vi "gfitsio-read-column-i32-scalar.vi"(7 "column":string, 8 "error in (no error)":errorcluster, 9 "row":i32, 11 "gfits refnum":T1) -> (0 "error out":errorcluster, 2 "data":i32, 3 "dup gfits refnum":T1)   [LabVIEW 2022 SP3, in "gfitsio.lvlib"]
doc: "Read elements from an ASCII or binary table column."
uses:
  gfitsio.lvlib
  gfitsio-refnum.ctl
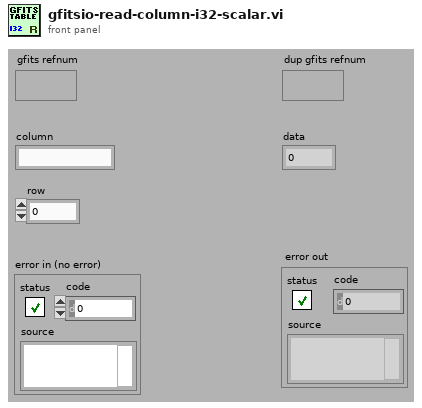
[diagram p1: front panel]
types:
  T1 = typedef "gfitsio.lvlib/gfitsio-refnum.ctl" = refnum<k1>
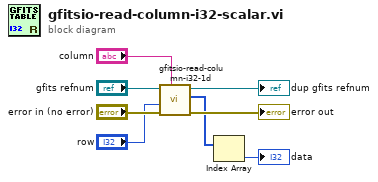
[diagram p0: block diagram]
diagram:
  n1 = call "gfitsio-read-column-i32-1d.vi"("column"="column", "error in (no error)"="error in (no error)", "row"="row", "gfits refnum"="gfits refnum") -> ("error out"=→"error out":errorcluster, "data"=w3:i32[], "dup gfits refnum"=→"dup gfits refnum":T1)  [unwired: 5 in]
  n2 = Index Array(array=w3) -> (element=→"data":i32)  [unwired: 1 in]
